vi "set bitrate adapting.vi"(8 "error in (no error)":errorcluster, 10 "enable (F)":bool, 11 "channel handle":u16 format="%x") -> (0 "error out":errorcluster)   [LabVIEW 2024, in "atsj peakcan basic.lvlib"]
uses:
  atsj peakcan basic.lvlib
  parameter.ctl
  set parameter - i32.vi
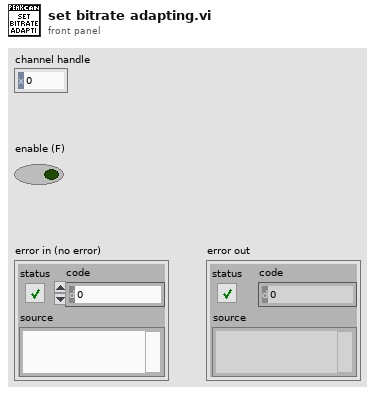
[diagram p1: front panel]
types:
  T1 = typedef "atsj peakcan basic.lvlib/parameter.ctl" = enum8{"DEVICE_ID", "5VOLTS_POWER", "RECEIVE_EVENT", "MESSAGE_FILTER", "API_VERSION", "CHANNEL_VERSION", "BUSOFF_AUTORESET", "LISTEN_ONLY", "LOG_LOCATION", "LOG_STATUS", "LOG_CONFIGURE", "LOG_TEXT", "CHANNEL_CONDITION", "HARDWARE_NAME", "RECEIVE_STATUS", "CONTROLLER_NUMBER", "TRACE_LOCATION", "TRACE_STATUS", "TRACE_SIZE", "TRACE_CONFIGURE", "CHANNEL_IDENTIFYING", "CHANNEL_FEATURES", "BITRATE_ADAPTING", "BITRATE_INFO", "BITRATE_INFO_FD", "BUSSPEED_NOMINAL", "BUSSPEED_DATA", "IP_ADDRESS", "LAN_SERVICE_STATUS", "ALLOW_STATUS_FRAMES", "ALLOW_RTR_FRAMES", "ALLOW_ERROR_FRAMES", "INTERFRAME_DELAY", "ACCEPTANCE_FILTER_11BIT", "ACCEPTANCE_FILTER_29BIT", "IO_DIGITAL_CONFIGURATION", "IO_DIGITAL_VALUE", "IO_DIGITAL_SET", "IO_DIGITAL_CLEAR", "IO_ANALOG_VALUE", "FIRMWARE_VERSION", "ATTACHED_CHANNELS_COUNT", "ATTACHED_CHANNELS", "ALLOW_ECHO_FRAMES", "DEVICE_PART_NUMBER", "HARD_RESET_STATUS", "LAN_CHANNEL_DIRECTION", "DEVICE_GUID"}
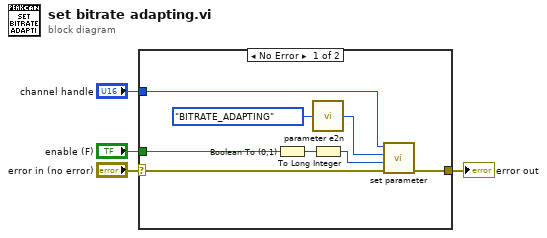
[diagram p0: block diagram]
diagram:
  n1 = case shown="No Error" "error in (no error)" {
    selector: "error in (no error)" -> [w10 w13]
    tunnel: [w9 w13] -> w3
    tunnel: "enable (F)" -> [w8 _]
    tunnel: "channel handle" -> [w5 _]
    frame No Error {
      n2 = Boolean To (0,1)(Boolean=w8) -> (0, 1=w7:i16)
      n3 = call "parameter e2n.vi"("parameter"=parameter."BITRATE_ADAPTING") -> ("number"=w11:u8)
      n4 = To Long Integer(number=w7) -> (32bit integer=w6:i32)
      n5 = call-poly "set parameter.vi"("error in (no error)"=w10, "value"=w6, "parameter"=w11, "channel"=w5) -> ("error out"=w9:errorcluster)  [unwired: 7 in]
    }
    frame Error {
    }
  }
  "error out" <- w3
